vi "ziExample-Module-DAQ_triggerUtility.vi"() -> ()   [LabVIEW 2009]
doc: "Control a Zurich instrument device via the LabOne Labview API. \nRequirements: Zurich Instruments MFLI, HF2 or UHFLI \nThis example shows how to start a DAQ trigger module and retrieve the Data.\n\n© Zurich Instruments AG, www.zhinst.com"
uses:
  <instrlib>/Zurich Instruments LabOne/Public/Modules/ziTypeModEnum.ctl
  <instrlib>/Zurich Instruments LabOne/Public/Modules/ziModSetValueBinary.vi
  <instrlib>/Zurich Instruments LabOne/Public/Configure/ziSetValueDoubleArray.vi
  <instrlib>/Zurich Instruments LabOne/Public/Modules/ziModSetValueDouble.vi
  <instrlib>/Zurich Instruments LabOne/Public/Modules/ziModGetDoubleData.vi
  <instrlib>/Zurich Instruments LabOne/Public/Utility/ziTicksToS_vector.vi
  <instrlib>/Zurich Instruments LabOne/Public/Utility/ziTicksToS_single.vi
  <instrlib>/Zurich Instruments LabOne/Zurich Instruments LabOne.lvlib
panel:
  in  "beating":bool caption="Beating (needs MD/MF Option)"
  out "Slide":dbl(slide) scale=0.0..1.0
  in  "subscribe":string="demods/0/sample.R.avg"
  out "Grid DEMOD X":dbl[][](graph)
  out "Error Out":errorcluster
  in  "stop":bool
  in  "run":bool caption="Run"
  in  "TriggerModulSetup":T1={"holdoff/time"=0.2, "holdoff/count"=0.0, "delay"=-0.00125, "duration"=0.01, "pulse/min"=0.0, "pulse/max"=0.0, "type"=1, "edge"=1, "count"=5.0, "bits"=1.0, "bitmask"=1.0, "triggernode"="demods/0/sample.R", "bandwidth"=0.0, "hysteresis"=0.003, "level"=0.03, "grid/mode"=1.0, "grid/cols"=100, "grid/rows"=100, "grid/direction"=0.0, "grid/repetitions"=1.0} {"grid/direction" items=["Forward", "Reverse", "Bi-directional"]; "grid/mode" items=["OFF", "Nearest", "Linear"]; "level" format="%#_6p"; "hysteresis" format="%#_6p"; "bandwidth" format="%#_6p"; "edge" items=["positive"=1, "negative"=2, "both"=3]; "type" items=["edge"=1, "digital"=2, "pulse"=3, "tracking edge"=4, "HW Trigger"=6, "tracking pulse"=7]}
  out "Demod X":T2(graph)
  in  "Address":string="DEV"
  out "Selected Device":string
  # "ziExample-Module-DAQ_triggerUtility.vi\nRequirements: \n- HF2LI, UHFLI or MFLI \n- MD Option\nsee block diagram for VI description"
  # "Tested Instruments:\n- HF2LI\n- UHFLI\n- MFLI"
  # "Trigger Settings"
  # "edge/pulse/tracking edge/tracking pulse"
  # "only for tracking mode"
  # "digital"
  # "Horizontal"
  # "only for pulse/tracking pulse"
  # "only for pulse/tracking pulse"
  # "Grid Mode"
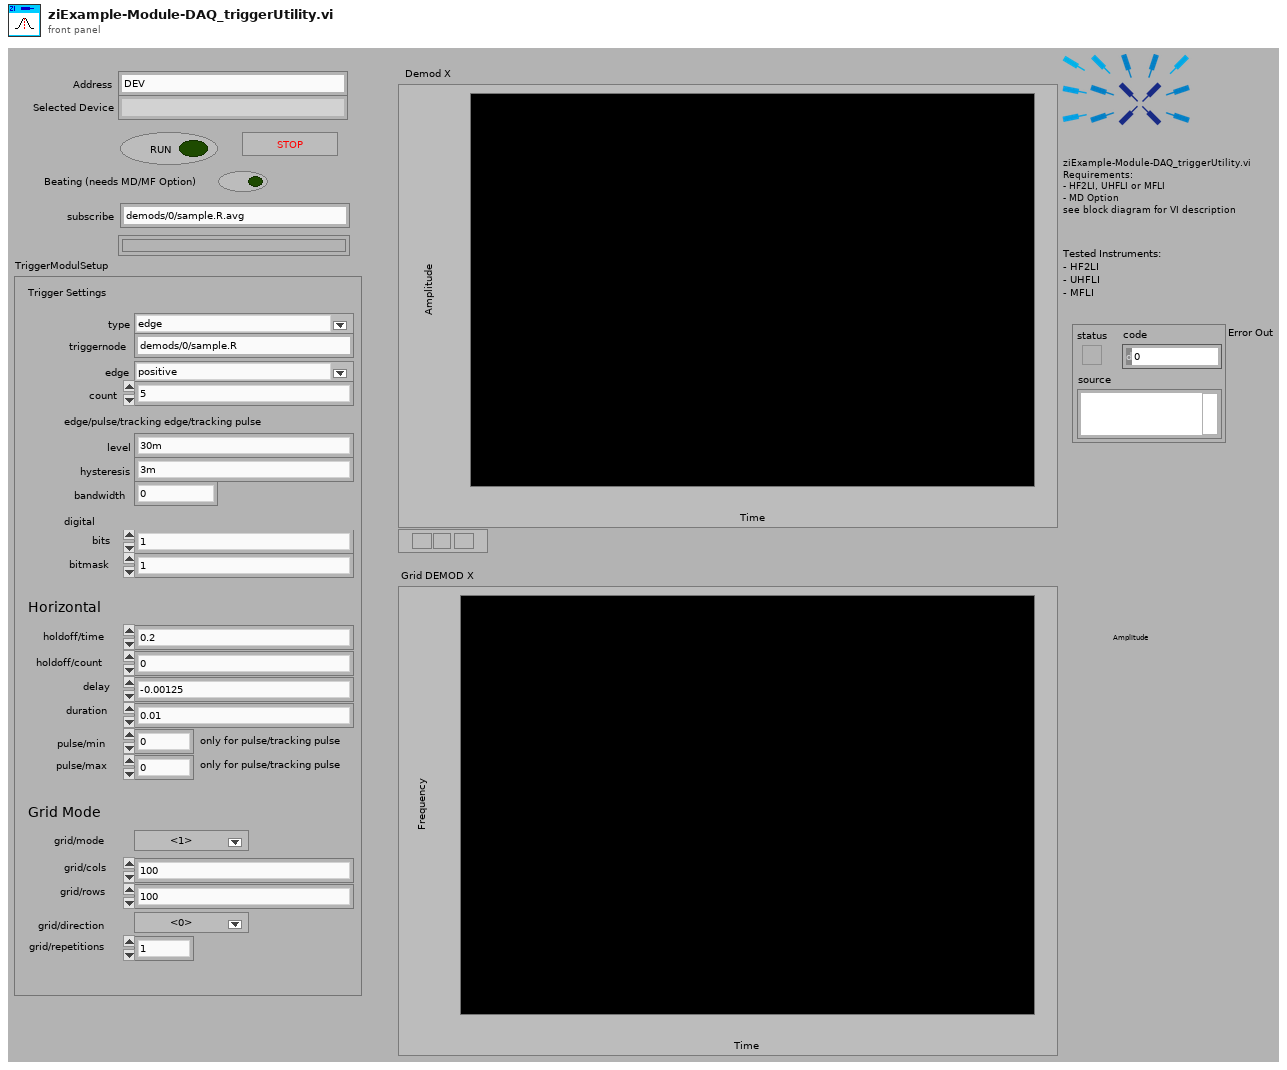
[diagram p1: front panel]
types:
  T1 = cluster{"holdoff/time":dbl, "holdoff/count":dbl, "delay":dbl, "duration":dbl, "pulse/min":dbl, "pulse/max":dbl, "type":u16, "edge":u16, "count":dbl, "bits":dbl, "bitmask":dbl, "triggernode":string, "bandwidth":dbl, "hysteresis":dbl, "level":dbl, "grid/mode":dbl, "grid/cols":u32, "grid/rows":u32, "grid/direction":dbl, "grid/repetitions":dbl}
  T2 = cluster{"Timestamp(s)":dbl[], "X (Vrms)":dbl[]}[]
  T3 = typedef "Zurich Instruments LabOne.lvlib/ziTypeModEnum.ctl" = u16
  T4 = typedef "Zurich Instruments LabOne.lvlib/ziTypeHandle.ctl" = cluster{"handleValid":bool, "Conn":u64, "Path Prefix":string, "Handle":u64, "Connected":bool, "Clockbase(s)":dbl}
  T5 = typedef "Zurich Instruments LabOne.lvlib/ziTypeModHandle.ctl" = cluster{"handleValid":bool, "Conn":u64, "ModHandle":u64, "moduleID":string, "Path Prefix":string}
  T6 = typedef "Zurich Instruments LabOne.lvlib/ziTypeModResults.ctl" = cluster{"PathArray":string[], "ValueType":T7, "NoOfResults":u64, "ziGenericHeader":T8[]}
  T7 = typedef "Zurich Instruments LabOne.lvlib/ziTypePollType.ctl" = enum16{"NONE", "DOUBLE_DATA", "INTEGER_DATA", "DEMOD_SAMPLE", "SCOPE_WAVE_HF2", "AUXIN_SAMPLE", "DIO_SAMPLE", "BYTE_ARRAY", "PWA_WAVE", "9", "10", "11", "12", "13", "14", "15", "TREE_CHANGE_DEPRI", "17", "ERROR", "19", "20", "21", "22", "23", "24", "25", "26", "27", "28", "29", "30", "31", "DOUBLE_DATA_TS", "INTEGER_DATA_TS", "34", "SCOPE_WAVE", "SCOPE_WAVE_EX", "37", "BYTE_ARRAY_TS", "39", "40", "41", "42", "43", "44", "45", "CNT_DATA", "47", "TREE_CHANGE", "49", "50", "51", "52", "53", "54", "55", "56", "57", "58", "59", "60", "61", "62", "63", "SWEEPER_DATA", "SPECTRUM_DATA", "ADVISOR_DATA", "VECTOR_DATA", "IMP_DATA"}
  T8 = typedef "Zurich Instruments LabOne.lvlib/ziTypeModGenericHeader.ctl" = cluster{"HeaderType":enum8{"HEADER_TYPE_NONE", "HEADER_TYPE_SWTRIGGER", "HEADER_TYPE_SWEEPER"}, "SampleFormat":u8, "SystemTime":timestamp, "CreatedTimeStamp":u64, "ChangedTimeStamp":u64, "Flags":u32, "ChunkSizeBytes":u64, "Name":string, "Status":u32, "GroupIndex":u32, "Color":u32, "ActiveRow":u32, "TriggerNumber":u64, "GridRows":u32, "GridCols":u32, "GridMode":u32, "GridOperation":u32, "GridDirection":u32, "GridRepetitions":u32, "GridColDelta":dbl, "GridColOffset":dbl, "GridRowDelta":dbl, "GridRowOffset":dbl, "Bandwidth":dbl, "Center":dbl, "Nenbw":dbl}
  T9 = typedef "Zurich Instruments LabOne.lvlib/ziTypeDoubleDataTSGrid.ctl" = cluster{"Timestamp (ticks)":u64[][], "Value":dbl[][]}
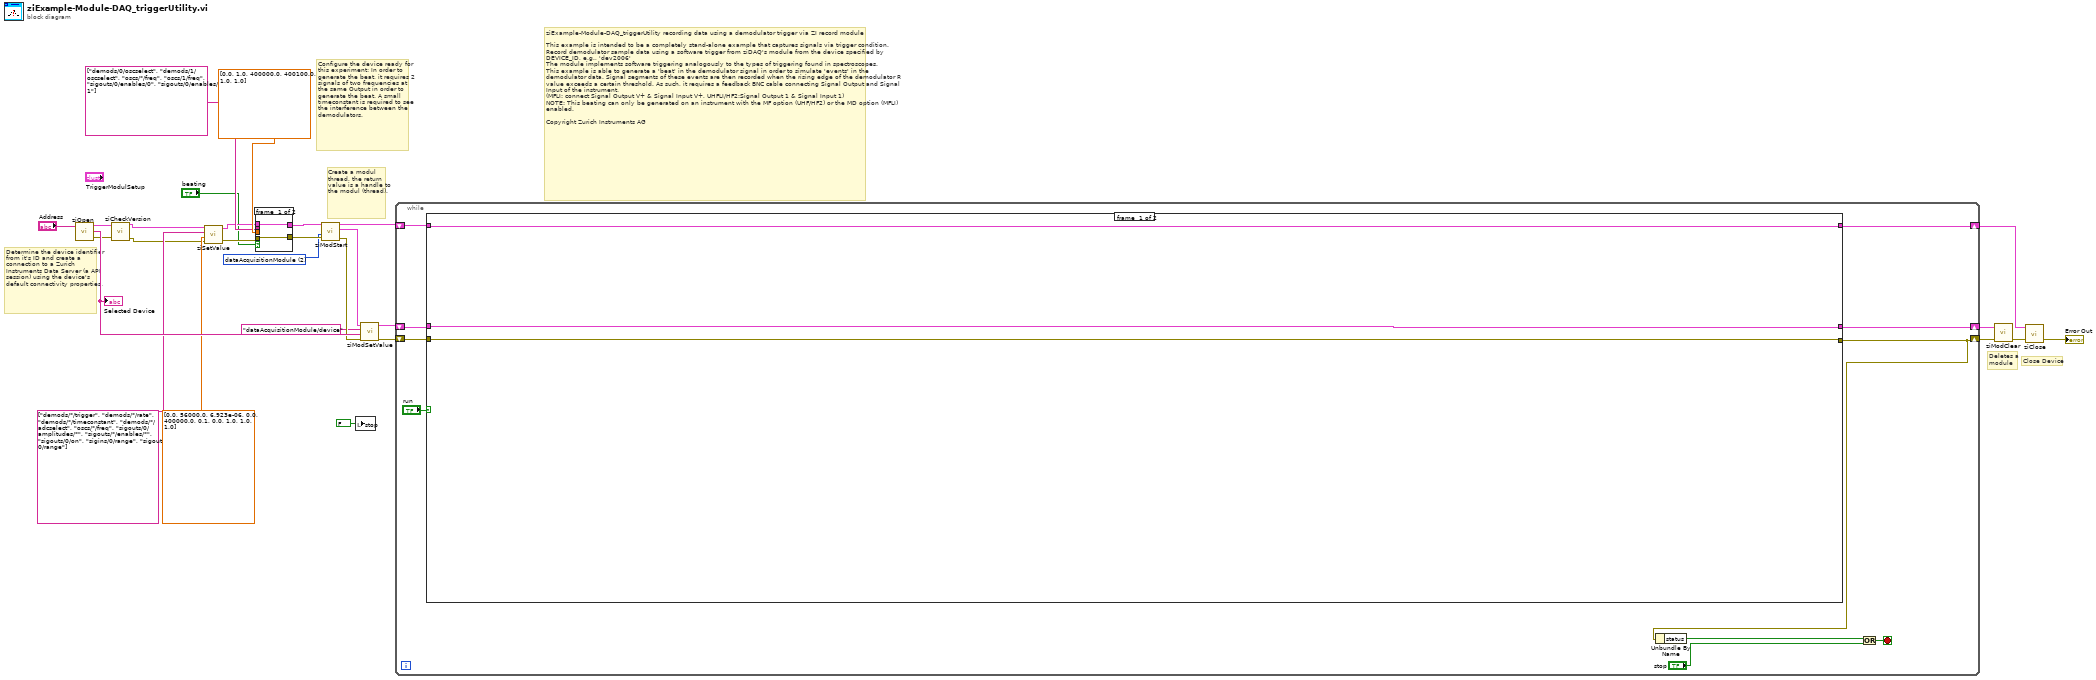
[diagram p0: block diagram]
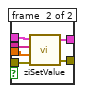
[diagram p2: hidden frame]
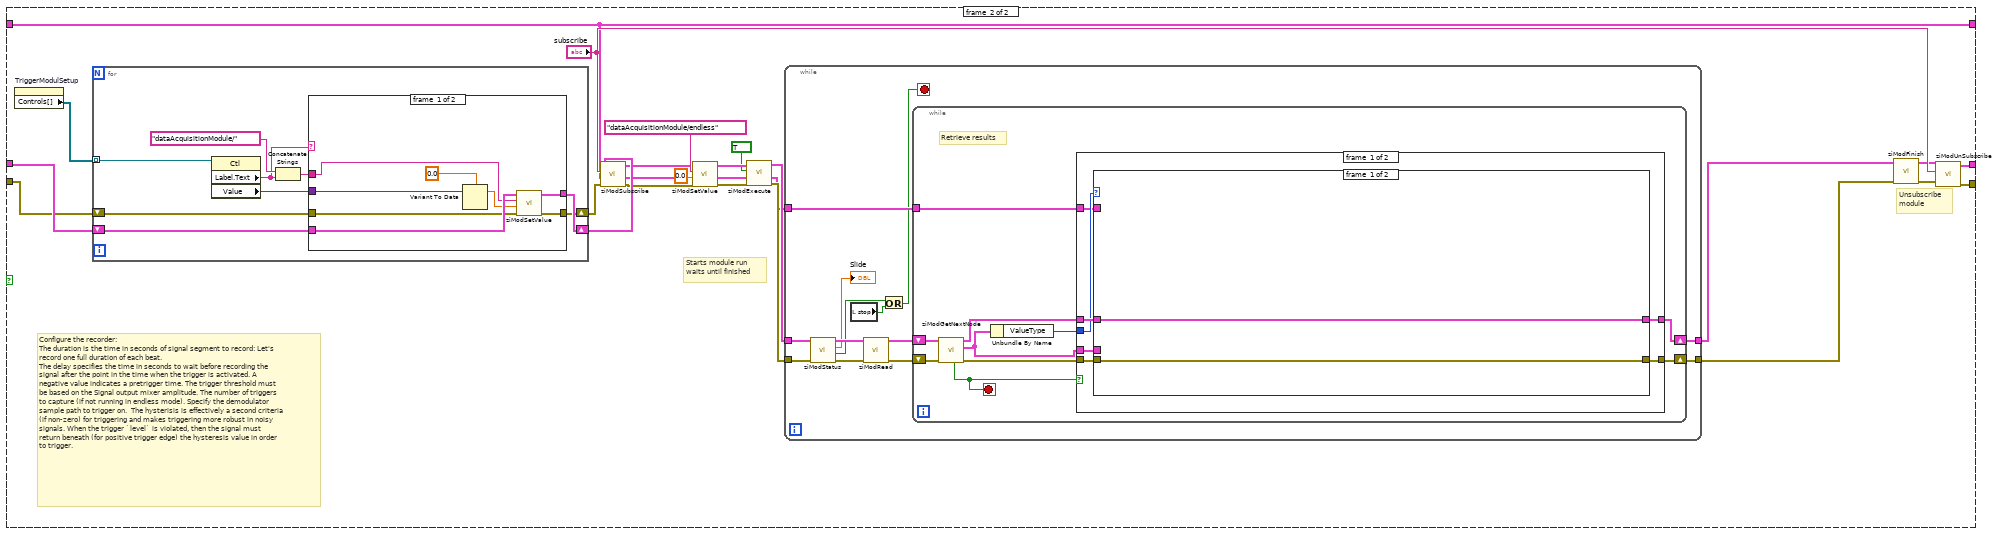
[diagram p3: hidden frame]
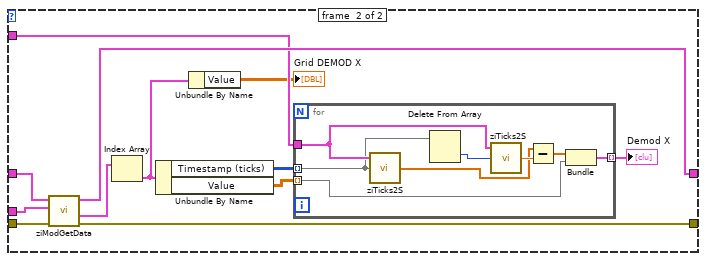
[diagram p4: hidden frame]
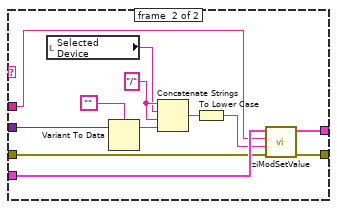
[diagram p6: hidden frame]
diagram:
  w1 = T3 2 items=["sweep", "scopeModule", "dataAcquisitionModule", "pidAdvisor", "awgModule", "impedanceModule", "multiDeviceSyncModule", "zoomFFT", "trigger", "deviceSettings", "record"] ("module Id")
  # "ziExample-Module-DAQ_triggerUtility recording data using a demodulator trigger via ZI record module\n\nThis example is intended to be a completely stand-alone example that captures signals via trigger condition. \nRecord demodulator sample data using a software trigger from ziDAQ's module from the device specified by DEVICE_ID, e.g., 'dev2006' \nThe module implements software triggering analogously to the types of triggering found in spectroscopes.\nThis example is able to generate a 'beat' in the demodulator signal in order to simulate 'events' in the demodulator data. Signal segments of these events are then recorded when the rising edge of the demodulator R value exceeds a certain threshold. As such, it requires a feedback BNC cable connecting Signal Output and Signal Input of the instrument. \n(MFLI: connect Signal Output V+ & Signal Input V+, UHFLI/HF2:Signal Output 1 & Signal Input 1)\nNOTE: This beating can only be generated on an instrument with the MF option (UHF/HF2) or the MD option (MFLI) enabled.\n\nCopyright Zurich Instruments AG"
  # "Configure the device ready for this experiment: In order to generate the beat, it requires 2 signals of two frequencies at the same Output in order to generate the beat. A small timeconstant is required to see the interference between the demodulators."
  # "Deletes a\nmodule"
  # "Create a modul thread, the return value is a handle to the modul (thread)."
  # "Close Device"
  # "Determine the device identifier from it's ID and create a connection to a Zurich Instruments Data Server (a API session) using the device's default connectivity properties."
  n1 = call <instrlib>:"ziOpen.vi"("Address"="Address") -> ("Error Out"=w4:errorcluster, "Selected Device"=w27:string, "HandleOut"=w5:T4)  [unwired: 1 in, 2 out]
  "Selected Device" <- w27
  n2 = call <instrlib>:"ziCheckVersion.vi"("Handle In"=w5, "Error In"=w4) -> ("Handle Out"=w3:T4, "Error Out"=w2:errorcluster)  [unwired: 11 in, 1 out]
  n3 = call-poly <instrlib>:"ziSetValue.vi"("Error In"=w2, "Values"=dbl[] [0.0, 56000.0, 6.923e-06, 0.0, 400000.0, 0.1, 0.0, 1.0, 1.0, 1.0], "Paths"=string[] ["demods/*/trigger", "demods/*/rate", "demods/*/timeconstant", "demods/*/adcselect", "oscs/*/freq", "sigouts/0/amplitudes/*", "sigouts/*/enables/*", "sigouts/0/on", "sigins/0/range", "sigouts/0/range"], "Handle In"=w3) -> ("Error Out"=w8:errorcluster, "Handle Out"=w9:T4)  [unwired: 1 in]
  n4 = case shown="False" "beating" {
    tunnel: [w30 w36] -> w23
    tunnel: [w29 w35] -> w22
    tunnel: string[] ["demods/0/oscselect", "demods/1/oscselect", "oscs/*/freq", "oscs/1/freq", "sigouts/0/enables/0", "sigouts/0/enables/1"] -> [_ w34]
    tunnel: dbl[] [0.0, 1.0, 400000.0, 400100.0, 1.0, 1.0] -> [_ w33]
    tunnel: w9 -> [w30 w32]
    tunnel: w8 -> [w29 w31]
    frame #0 {
    }
    frame #1 {
      n5 = call-poly <instrlib>:"ziSetValue.vi"("Error In"=w31, "Values"=w33, "Paths"=w34, "Handle In"=w32) -> ("Error Out"=w35:errorcluster, "Handle Out"=w36:T4)  [unwired: 1 in]
    }
  }
  n6 = call <instrlib>:"ziModStart.vi"("Error In"=w22, "module Id"=w1, "Handle In"=w23) -> ("Error Out"=w25:errorcluster, "ModHandle Out"=w26:T5, "Handle Out"=w19:T4)  [unwired: 6 in]
  n7 = local write "stop"(FALSE ("stop")) -> ()
  n8 = call-poly <instrlib>:"ziModSetValue.vi"("Error In"=w25, "Data"=w27, "Path"="dataAcquisitionModule/device", "ModHandle In"=w26) -> ("Error Out"=w20:errorcluster, "ModHandle Out"=w15:T5)  [unwired: 6 in]
  n9 = while {
    shift-right: [w42] -> w17
    shift-left: w15 -> [w45]
    shift-right: [w37] -> w18
    shift-left: w20 -> [w44]
    shift-right: [w41] -> w6
    shift-left: w19 -> [w46]
    stop <- w38 stop-if-true
    n10 = case shown="True" "run" {
      tunnel: [w48 w62] -> w42
      tunnel: [w49 w52] -> w37
      tunnel: w46 -> [w47 w53]
      tunnel: w45 -> [w48 w66]
      tunnel: w44 -> [w49 w65]
      tunnel: [w47 w53] -> w41
      frame #0 {
      }
      frame #1 {
        # "Unsubscribe\nmodule"
        # "Starts module run\nwaits until finished"
        # "Configure the recorder:\nThe duration is the time in seconds of signal segment to record: Let's record one full duration of each beat.\nThe delay specifies the time in seconds to wait before recording the signal after the point in the time when the trigger is activated. A negative value indicates a pretrigger time. The trigger threshold must be based on the Signal output mixer amplitude. The number of triggers to capture (if not running in endless mode). Specify the demodulator sample path to trigger on.  The hysterisis is effectively a second criteria (if non-zero) for triggering and makes triggering more robust in noisy signals. When the trigger `level` is violated, then the signal must return beneath (for positive trigger edge) the hysteresis value in order to trigger."
        n11 = property on="TriggerModulSetup" class="Clust (strict)"() -> ("Controls[]"=w69:refnum<vi>[])  [unwired: 2 in, 2 out]
        n12 = for {
          tunnel: w69 -> [w134] mode=indexing
          shift-right: [w131] -> w67
          shift-left: w65 -> [w129]
          shift-right: [w132] -> w68
          shift-left: w66 -> [w130]
          n13 = property class="Ctl"(reference=w134) -> ("Label.Text"=w127:string, "Value"=w126:variant)  [unwired: 1 in, 2 out]
          n14 = Concatenate Strings("dataAcquisitionModule/" ("string"), w127) -> (w128:string)
          n15 = case shown="\"triggernode\"" w127 {
            tunnel: w128 -> [w135 w148]
            tunnel: w126 -> [w142 w153]
            tunnel: [w139 w152] -> w132
            tunnel: [w138 w151] -> w131
            tunnel: w130 -> [w140 w150]
            tunnel: w129 -> [w137 w149]
            frame #0 {
              n16 = Variant To Data(Variant=w142, type=0.0) -> (data=w136:dbl)  [unwired: 1 in, 1 out]
              n17 = call-poly <instrlib>:"ziModSetValue.vi"("Error In"=w137, "Value"=w136, "Path"=w135, "ModHandle In"=w140) -> ("Error Out"=w138:errorcluster, "ModHandle Out"=w139:T5)  [unwired: 6 in]
            }
            frame #1 {
              w147 = "/"
              n18 = local read "Selected Device"() -> (w146:string)
              n19 = Variant To Data(Variant=w153, type="") -> (data=w145:string)  [unwired: 1 in, 1 out]
              n20 = Concatenate Strings(w147, w146, w147, w145) -> (w144:string)
              n21 = To Lower Case(string=w144) -> (all lower case string=w143:string)
              n22 = call-poly <instrlib>:"ziModSetValue.vi"("Error In"=w149, "Data"=w143, "Path"=w148, "ModHandle In"=w150) -> ("Error Out"=w151:errorcluster, "ModHandle Out"=w152:T5)  [unwired: 6 in]
            }
          }
        }
        n23 = call <instrlib>:"ziModSubscribe.vi"("Error In"=w67, "Path"="subscribe", "ModHandle In"=w68) -> ("Error Out"=w51:errorcluster, "ModHandle Out"=w50:T5)  [unwired: 6 in]
        n24 = call-poly <instrlib>:"ziModSetValue.vi"("Error In"=w51, "Value"=0.0, "Path"="dataAcquisitionModule/endless", "ModHandle In"=w50) -> ("Error Out"=w63:errorcluster, "ModHandle Out"=w64:T5)  [unwired: 6 in]
        n25 = call <instrlib>:"ziModExecute.vi"("Error In"=w63, "Modal (F)"=TRUE, "ziModHandle In"=w64) -> ("Error Out"=w58:errorcluster, "ziModHandle Out"=w59:T5)  [unwired: 5 in, 1 out]
        n26 = while {
          tunnel: w53 -> [w84]
          tunnel: w59 -> [w79]
          tunnel: w58 -> [w78]
          tunnel: [w77] -> w56
          tunnel: [w76] -> w55
          stop <- w72 stop-if-true
          n27 = call <instrlib>:"ziModStatus.vi"("Error In"=w78, "ModHandle IN"=w79) -> ("Error Out"=w80:errorcluster, "Finished?"=w73:bool, "Progress (unity)"=→"Slide":dbl, "ModHandle Out"=w81:T5)  [unwired: 5 in]
          n28 = local read "stop"() -> (w74:bool)
          n29 = call <instrlib>:"ziModRead.vi"("error in"=w80, "ziModHandle In"=w81) -> ("error out"=w83:errorcluster, "ziModHandle Out"=w82:T5)  [unwired: 8 in]
          n30 = Or(x=w73, y=w74) -> (x .or. y?=w72:bool)
          n31 = while {
            shift-right: [w89] -> w76
            shift-left: w82 -> [w93]
            shift-right: [w90] -> w77
            shift-left: w83 -> [w94]
            tunnel: w84 -> [w88]
            stop <- w87 stop-if-true
            # "Retrieve results"
            n32 = call <instrlib>:"ziModGetNextNode.vi"("Error In"=w94, "ModHandle In"=w93) -> ("Error Out"=w91:errorcluster, "ModResults"=w85:T6, "ModHandle Out"=w92:T5, "NoData"=w87:bool)  [unwired: 6 in]
            n33 = Unbundle By Name(w85) -> ("ValueType"=w86:T7)
            n34 = case shown="False" w87 {
              tunnel: w85 -> [w101 _]
              tunnel: w92 -> [w100 w125]
              tunnel: w91 -> [w99 w124]
              tunnel: [w98 w124] -> w90
              tunnel: [w97 w125] -> w89
              tunnel: w86 -> [w96 _]
              tunnel: w88 -> [w95 _]
              frame #0 {
                n35 = case shown="\"DOUBLE_DATA_TS\"" w96 {
                  tunnel: w100 -> [w103 w108]
                  tunnel: w101 -> [_ w107]
                  tunnel: w99 -> [w102 w112]
                  tunnel: [w102 w113] -> w98
                  tunnel: [w103 w115] -> w97
                  tunnel: w95 -> [_ w114]
                  frame #0 {
                  }
                  frame #1 {
                    n36 = call-poly <instrlib>:"ziModGetData.vi"("Error In"=w112, "ModResults"=w107, "ModHandle In"=w108) -> ("Error Out"=w113:errorcluster, "DoubleSampleGrid"=w111:T9[], "ModHandle Out"=w115:T5)  [unwired: 4 in, 2 out]
                    n37 = Index Array(array=w111) -> (element=w106:T9)  [unwired: 1 in]
                    n38 = Unbundle By Name(w106) -> ("Timestamp (ticks)"=w105:u64[][], "Value"=w104:dbl[][])
                    n39 = Unbundle By Name(w106) -> ("Value"=→"Grid DEMOD X":dbl[][])
                    n40 = for {
                      tunnel: [w123] -> w109 mode=indexing
                      tunnel: w114 -> [w122]
                      tunnel: w105 -> [w117] mode=indexing
                      tunnel: w104 -> [w118] mode=indexing
                      n41 = call-poly <instrlib>:"ziTicks2S.vi"("Timestamp (ticks)"=w117, "Handle In"=w122) -> ("Timestamp(s)"=w120:dbl[])  [unwired: 1 in, 2 out]
                      n42 = Delete From Array(array=w117) -> (deleted portion=w116:u64)  [unwired: 2 in, 1 out]
                      n43 = call-poly <instrlib>:"ziTicks2S.vi"("Timestamp(ticks)"=w116, "Handle In"=w122) -> ("Timestamp(s)"=w121:dbl)  [unwired: 1 in, 2 out]
                      n44 = Subtract(x=w120, y=w121) -> (x-y=w119:dbl[])
                      n45 = Bundle(w119, "Value"=w118) -> (w123:cluster{dbl[], "Value":dbl[]})  [unwired: 1 in]
                    }
                    "Demod X" <- w109
                  }
                }
              }
              frame #1 {
              }
            }
          }
        }
        n46 = call <instrlib>:"ziModFinish.vi"("Error In"=w56, "ziModHandle In"=w55) -> ("Error Out"=w57:errorcluster, "ziModHandle Out"=w54:T5)  [unwired: 7 in]
        n47 = call <instrlib>:"ziModUnSubscribe.vi"("Error In"=w57, "Path (\"/\")"="subscribe", "ModHandle In"=w54) -> ("Error Out"=w52:errorcluster, "ModHandle Out"=w62:T5)  [unwired: 7 in]
      }
    }
    n48 = Unbundle By Name(w37) -> ("status"=w40:bool)
    n49 = Or(x=w40, y="stop") -> (x .or. y?=w38:bool)
  }
  n50 = call <instrlib>:"ziModClear.vi"("Error In"=w18, "ziModHandle In"=w17) -> ("Error Out"=w28:errorcluster)  [unwired: 7 in, 1 out]
  n51 = call <instrlib>:"ziClose.vi"("Error In"=w28, "Handle In"=w6) -> ("Error Out"=→"Error Out":errorcluster)  [unwired: 2 in, 1 out]
